vi "Measurement to Protocol Settings.vi"(11 "Measurement Configuration":T1 {"Settling time" min=0.0 max=5.0 step=0.0001 format="%.3f"; "Settling cycles" min=0 max=100 step=1}) -> (3 "Protocol settings":T2)   [LabVIEW 2021, in "audio adc shared.lvlib"]
uses:
  controls/Protocol Settings.ctl
  frequency response/Frequency Response_Audio ADC/Measurement Configuration.ctl
  audio adc shared.lvlib
  controls/audio adc controls.lvlib
  frequency response/Frequency Response_Audio ADC/Frequency Response_Audio ADC.lvlib
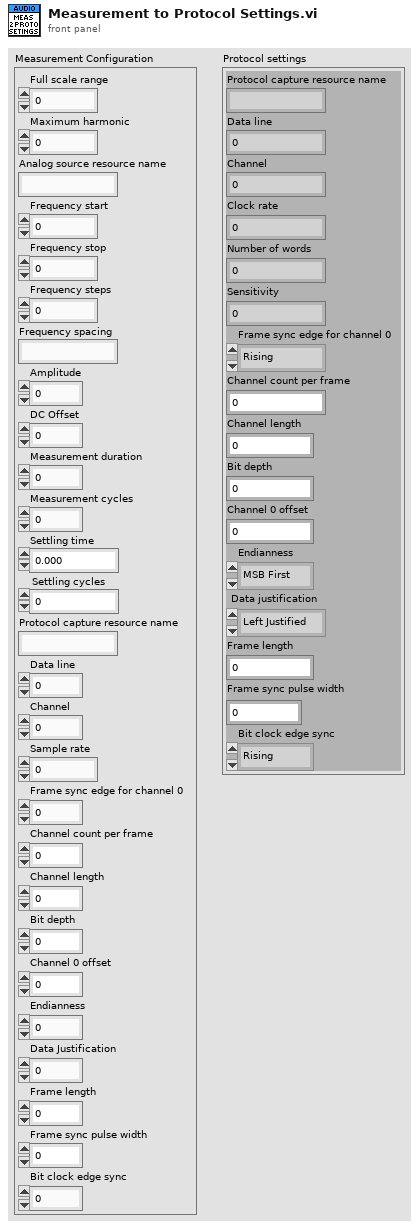
[diagram p1: front panel]
types:
  T1 = typedef "Frequency Response_Audio ADC.lvlib/Measurement Configuration.ctl" = cluster{"Full scale range":dbl, "Maximum harmonic":i32, "Analog source resource name":string, "Frequency start":dbl, "Frequency stop":dbl, "Frequency steps":i32, "Frequency spacing":string, "Amplitude":dbl, "DC Offset":dbl, "Measurement duration":dbl, "Measurement cycles":i32, "Settling time":dbl, "Settling cycles":i32, "Protocol capture resource name":string, "Data line":u16, "Channel":u32, "Sample rate":dbl, "Frame sync edge for channel 0":u32, "Channel count per frame":u32, "Channel length":u32, "Bit depth":u32, "Channel 0 offset":u32, "Endianness":u32, "Data justification":u32, "Frame length":u32, "Frame sync pulse width":u32, "Bit clock edge sync":u32}
  T2 = typedef "audio adc controls.lvlib/Protocol Settings.ctl" = cluster{"Protocol capture resource name":string, "Data line":u16, "Channel":u32, "Clock rate":u32, "Number of words":i32, "Sensitivity":dbl, "Frame sync edge for channel 0":enum32{"Rising", "Falling"}, "Channel count per frame":u8, "Channel length":u16, "Bit depth":u8, "Channel 0 offset":u16, "Endianness":enum32{"MSB First", "LSB First"}, "Data justification":enum32{"Left Justified", "Right Justified"}, "Frame length":u16, "Frame sync pulse width":u16, "Bit clock edge sync":enum32{"Rising", "Falling"}}
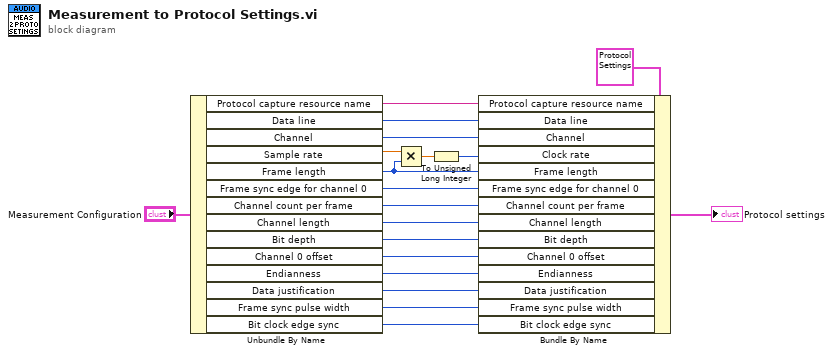
[diagram p0: block diagram]
diagram:
  n1 = Unbundle By Name("Measurement Configuration") -> ("Protocol capture resource name"=w16:string, "Data line"=w17:u16, "Channel"=w18:u32, "Sample rate"=w2:dbl, "Frame length"=w3:u32, "Frame sync edge for channel 0"=w13:u32, "Channel count per frame"=w12:u32, "Channel length"=w11:u32, "Bit depth"=w10:u32, "Channel 0 offset"=w9:u32, "Endianness"=w8:u32, "Data justification"=w7:u32, "Frame sync pulse width"=w6:u32, "Bit clock edge sync"=w5:u32)
  n2 = Multiply(x=w2, y=w3) -> (x*y=w4:dbl)
  n3 = To Unsigned Long Integer(number=w4) -> (unsigned 32bit integer=w1:u32)
  n4 = Bundle By Name(cluster=T2 {"Protocol capture resource name"="", "Data line"=0, "Channel"=0, "Clock rate"=12288000, "Number of words"=19200, "Sensitivity"=0.34762, "Frame sync edge for channel 0"=enum."Falling", "Channel count per frame"=2, "Channel length"=32, "Bit depth"=24, "Channel 0 offset"=1, "Endianness"=enum."MSB First", "Data justification"=enum."Left Justified", "Frame length"=64, "Frame sync pulse width"=32, "Bit clock edge sync"=enum."Falling"} ("Protocol settings"), "Protocol capture resource name"=w16, "Data line"=w17, "Channel"=w18, "Clock rate"=w1, "Frame length"=w3, "Frame sync edge for channel 0"=w13, "Channel count per frame"=w12, "Channel length"=w11, "Bit depth"=w10, "Channel 0 offset"=w9, "Endianness"=w8, "Data justification"=w7, "Frame sync pulse width"=w6, "Bit clock edge sync"=w5) -> (→"Protocol settings":T2)
